vi "Convertir des °C en °F.vi"(1 "cilcius":dbl) -> (0 "Fah":dbl)   [LabVIEW 2014]
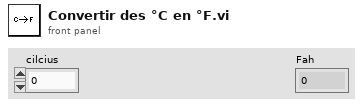
[diagram p1: front panel]
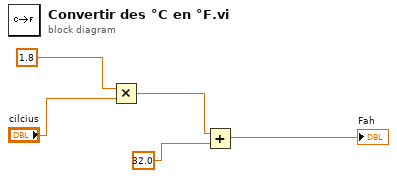
[diagram p0: block diagram]
diagram:
  n1 = Multiply(x=1.8, y="cilcius") -> (x*y=w2:dbl)
  n2 = Add(x=w2, y=32.0) -> (x+y=→"Fah":dbl)
